vi "RSZVB Get Virtual Transform Single Ended Port.vi"(4 "Physical Port Number (1)":i32=1, 5 "Circuit Model (1: Serial C, shunt L)":i32(ring)=1 items=["Serial C, shunt L"=1, "Serial L, shunt C"=2, "Serial C, shunt C"=3, "Serial L, shunt L"=4, "Shunt L, serial C"=5, "Shunt C, serial L"=6, "Shunt C, serial C"=7, "Shunt L, serial L"=8], 6 "Parameter Number (1)":i32=1, 7 "Parameter Type (0: Capacitance)":i32(ring) items=["Capacitance", "Inductance", "Resistance"], 8 "error in (no error)":errorcluster {"code" format="%.0x"}, 9 "Function Type (0: Deembedding)":i32(ring) items=["Deembedding", "Embedding"], 10 "Channel (1)":i32=1, 11 "VISA session":refnum<visa-resource-name>) -> (0 "error out":errorcluster {"code" format="%.0x"}, 2 "Value":dbl format="%^.3e", 3 "dup VISA session":refnum<visa-resource-name>)   [LabVIEW 2011]
doc: "This VI returns the capacitance, inductance or resistance values C1, C2, L1, L2 or R1, R2 in the different circuit models for single ended port deembedding/embedding.\n\nRemote-control command(s):\nCALCulate<Ch>:TRANsform:VNETworks:SENDed:DEEMbedding<Ph_pt>:PARameters:C<no>? CSL | LSC | CSC | SLC | SCL | SCC\nCALCulate<Ch>:TRANsform:VNETworks:SENDed:DEEMbedding<Ph_pt>:PARameters:L<no>? CSL | LSC | LSL | SLC | SCL | SLL\nCALCulate<Ch>:TRANsform:VNETworks:SENDed:DEEMbedding<Ph_pt>:PARameters:R<no>? CSL | LSC | CSC | LSL | SLC | SCL | SCC | SLL\nCALCulate<Ch>:TRANsform:VNETworks:SENDed:EMBedding<Ph_pt>:PARameters:C<no> CSL? | LSC | CSC | SLC | SCL | SCC\nCALCulate<Ch>:TRANsform:VNETworks:SENDed:EMBedding<Ph_pt>:PARameters:L<no> CSL? | LSC | LSL | SLC | SCL | SLL\nCALCulate<Ch>:TRANsform:VNETworks:SENDed:EMBedding<Ph_pt>:PARameters:R<no> CSL? | LSC | CSC | LSL | SLC | SCL | SCC | SLL"
uses:
  _utility/RSZVB Global Data.vi
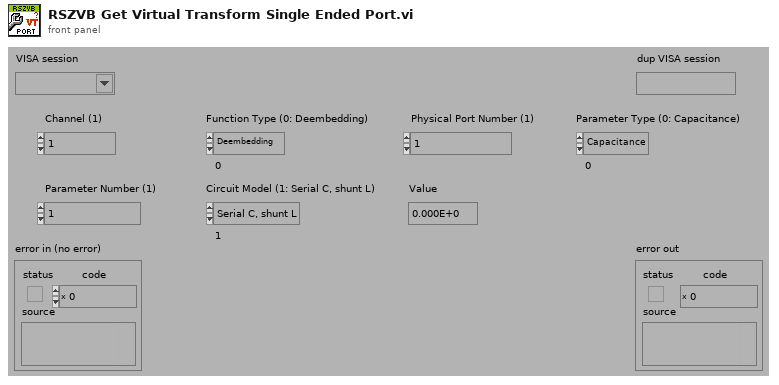
[diagram p1: front panel]
types:
  T1 = cluster{"Error Checking (T: On)":bool, "Installed Options":string[], "Data Valid?":bool, "Ports":i32, "Model":string[], "Option Checking (T: On)":bool}[]
  T2 = cluster{"Error Checking (T: On)":bool, "Installed Options":string[], "Data Valid?":bool, "Ports":i32, "Model":string[], "Option Checking (T: On)":bool}
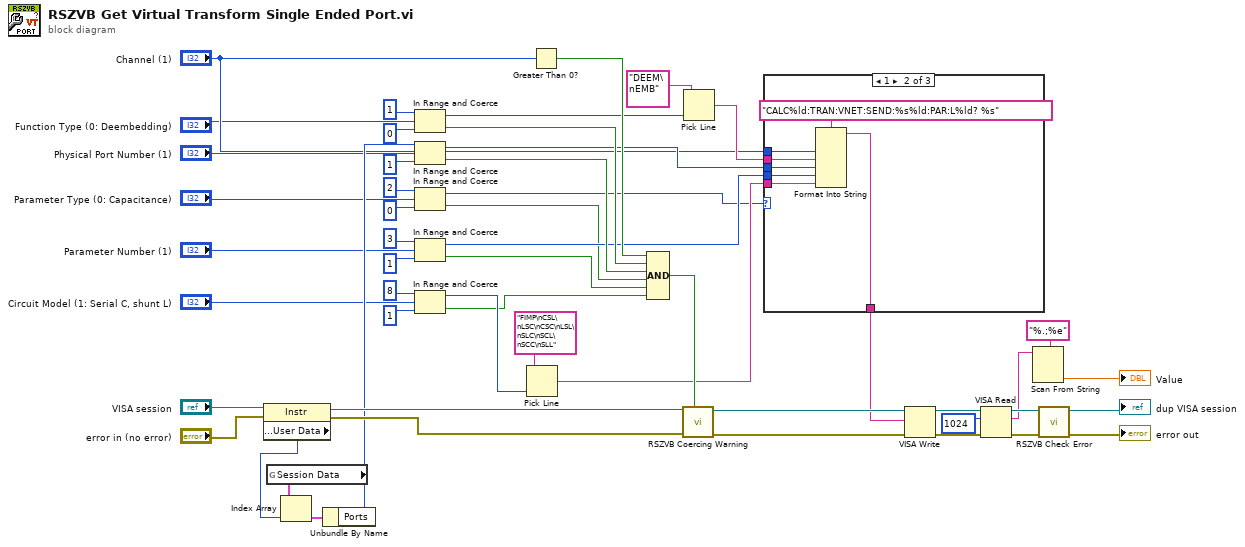
[diagram p0: block diagram]
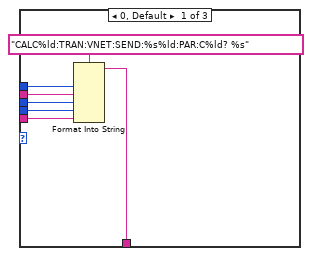
[diagram p2: hidden frame]
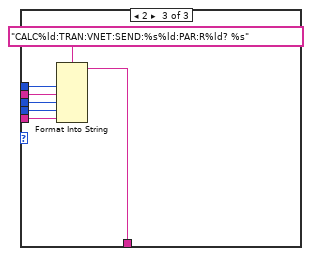
[diagram p3: hidden frame]
diagram:
  n1 = property class="Instr"(reference="VISA session", error in="error in (no error)") -> (reference out=w49:refnum<visa-resource-name>, error out=w50:errorcluster, "General Settings:User Data"=w20:u32)
  n2 = global read "RSZVB Global Data.vi" "Session Data"() -> (w23:T1)
  n3 = Index Array(array=w23, index=w20) -> (element=w22:T2)
  n4 = Unbundle By Name(w22) -> ("Ports"=w21:i32)
  n5 = In Range and Coerce(upper limit=1 ("lower limit"), x="Function Type (0: Deembedding)", lower limit=0) -> (coerced(x)=w40:i32, In Range?=w43:bool)
  n6 = In Range and Coerce(upper limit=w21, x="Physical Port Number (1)", lower limit=1) -> (coerced(x)=w42:i32, In Range?=w38:bool)
  n7 = In Range and Coerce(upper limit=2 ("lower limit"), x="Parameter Type (0: Capacitance)", lower limit=0) -> (coerced(x)=w24:i32, In Range?=w27:bool)
  n8 = In Range and Coerce(upper limit=3 ("lower limit"), x="Parameter Number (1)", lower limit=1) -> (coerced(x)=w28:i32, In Range?=w26:bool)
  n9 = In Range and Coerce(upper limit=8 ("lower limit"), x="Circuit Model (1: Serial C, shunt L)", lower limit=1) -> (coerced(x)=w30:i32, In Range?=w25:bool)
  n10 = Pick Line(multi-line string="FIMP\nCSL\nLSC\nCSC\nLSL\nSLC\nSCL\nSCC\nSLL", line index=w30) -> (output string=w29:string)  [unwired: 1 in]
  n11 = Greater Than 0?(x="Channel (1)") -> (x > 0?=w46:bool)
  n12 = Compound Arithmetic op=AND(w46, w43, w38, w27, w26, w25) -> (w45:bool)
  n13 = call "RSZVB Coercing Warning.vi"("In Range?"=w45, "error in (no error)"=w50, "VISA session"=w49) -> ("error out"=w51:errorcluster, "dup VISA session"=w52:refnum<visa-resource-name>)  [unwired: 7 in]
  n14 = Pick Line(multi-line string="DEEM\nEMB", line index=w40) -> (output string=w39:string)  [unwired: 1 in]
  n15 = case shown="1" w24 {
    tunnel: "Channel (1)" -> [w58 w65 w72]
    tunnel: w42 -> [w56 w63 w70]
    tunnel: w39 -> [w57 w64 w71]
    tunnel: w29 -> [w55 w61 w68]
    tunnel: w28 -> [w54 w62 w69]
    tunnel: [w53 w60 w67] -> w19
    frame 0, Default {
      n16 = Format Into String(format string="CALC%ld:TRAN:VNET:SEND:%s%ld:PAR:C%ld? %s", w58, w57, w56, w54, w55) -> (resulting string=w53:string)  [unwired: 2 in, 1 out]
    }
    frame 1 {
      n17 = Format Into String(format string="CALC%ld:TRAN:VNET:SEND:%s%ld:PAR:L%ld? %s", w65, w64, w63, w62, w61) -> (resulting string=w60:string)  [unwired: 2 in, 1 out]
    }
    frame 2 {
      n18 = Format Into String(format string="CALC%ld:TRAN:VNET:SEND:%s%ld:PAR:R%ld? %s", w72, w71, w70, w69, w68) -> (resulting string=w67:string)  [unwired: 2 in, 1 out]
    }
  }
  n19 = VISA Write(VISA resource name=w52, write buffer=w19, error in (no error)=w51) -> (VISA resource name out=w12:refnum<visa-resource-name>, error out=w13:errorcluster)  [unwired: 1 out]
  n20 = VISA Read(VISA resource name=w12, byte count=u32 1024 ("byte count (0)"), error in (no error)=w13) -> (VISA resource name out=w17:refnum<visa-resource-name>, read buffer=w14:string, error out=w16:errorcluster)  [unwired: 1 out]
  n21 = Scan From String(format string="%.;%e", input string=w14) -> (output 1=→"Value":dbl)  [unwired: 3 in, 3 out]
  n22 = call "RSZVB Check Error.vi"("error in (no error)"=w16, "VISA session"=w17) -> ("error out"=→"error out":errorcluster, "dup VISA session"=→"dup VISA session":refnum<visa-resource-name>)  [unwired: 8 in]
